vi "Scripting_AlignToConnectorPane.vi"(8 "error in (no error)":errorcluster, 11 "VI Ref":refnum<vi>) -> (0 "error out":errorcluster)   [LabVIEW 2020, in "Scripting.lvclass"]
doc: "This VI arranges the Front Panel objects to match the Connector Pane layout"
uses:
  Scripting.lvclass
panel:
  # "Do not change the connector pane of this VI.\n\nSee the block diagram for directions on how to use this template."
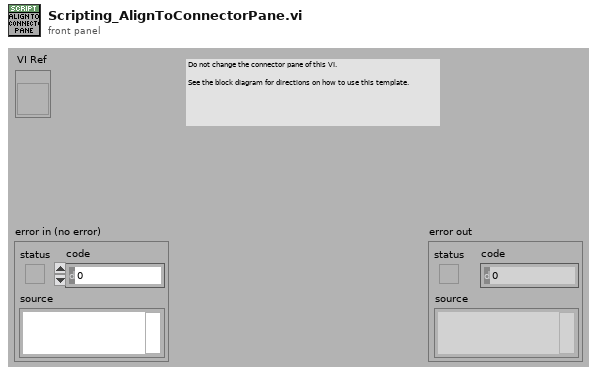
[diagram p1: front panel]
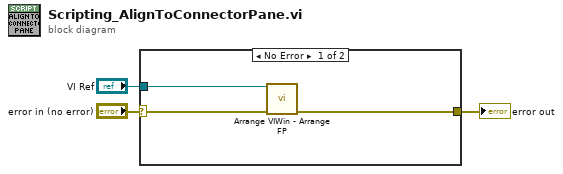
[diagram p0: block diagram]
diagram:
  n1 = case shown="No Error" "error in (no error)" {
    selector: "error in (no error)" -> [w5 w7]
    tunnel: [w4 w7] -> w2
    tunnel: "VI Ref" -> [w6 _]
    frame No Error {
      n2 = call <resource>:"Arrange VIWin - Arrange FP.vi"("VI"=w6, "error in"=w5) -> ("error out"=w4:errorcluster)  [unwired: 13 in]
    }
    frame Error {
    }
  }
  "error out" <- w2
